vi "Configure Standard Waveform.vi"(0 "VISA resource name":refnum<visa-resource-name>, 1 "Amplitude (0.1 Vpp)":dbl=0.1, 2 "Phase Angle (0 Degree)":dbl, 5 "Channel (1: 1)":i32(ring)=1 items=["1"=1, "2"=2], 7 "Waveform Function (0: Sine)":i32(ring) items=["Sine"=0, "Square"=1, "Ramp"=2, "Noise"=3, "DC"=4, "Triangle"=5, "Pulse"=6, "Sinc"=11, "D-Lorentz"=12, "Gaussian"=13, "Expo Fall"=14, "Expo Rise"=15, "Haversine"=16], 9 "Frequency/Sample Rate/Bandwidth (1000 Hz)":dbl=1000.0 format="%#.4f", 11 "error in (no error)":errorcluster, 12 "Amplitude Unit (0: Vpp)":i32(ring) items=["Vpp", "VRMS", "DBM"], 13 "Angle Unit (0: Degree)":i32(ring) items=["Degree", "Radian", "Second"], 14 "DC Offset (0 V)":dbl) -> (4 "VISA resource name out":refnum<visa-resource-name>, 15 "error out":errorcluster)   [LabVIEW 2020, in "Agilent 3352X Series.lvlib"]
doc: "Selects a standard waveform and configure the frequency/sample rate, amplitude, offset, and phase for it.\nStandard waveform includes Sine, Square, Ramp, Noise, DC, Triangle, Sinc, D-Lorentz, Gaussian, Expo Fall, Expo Rise and Haversine\nUse Configure PRBS Waveform.vi to configure PRBS waves; use Configure Pulse Waveform.vi to configure Pulse waves.\nUse Configure Standard Waveform Advanced (Ramp) VI to set ramp symmetry for ramp wave; use Configure Standard Waveform Advanced (Suqare) VI to set duty cycle for square wave.\n<b>Note</b>:\n(1). Using this vi will automatically turn off sweep and switch to fixed frequency mode.\n(2). When select Sinc, D-Lorentz, Gaussian, Expo Fall, Expo Rise and HaverSine, a system owned Arbitrary wave is loaded and you can do arbitrary wave related settings like Filter mode and Advance mode use Configure Arbitrary Waveform (Advanced).vi"
uses:
  Agilent 3352X Series.lvlib
panel:
  # "Amplitude Settings"
  # "Phase Settings"
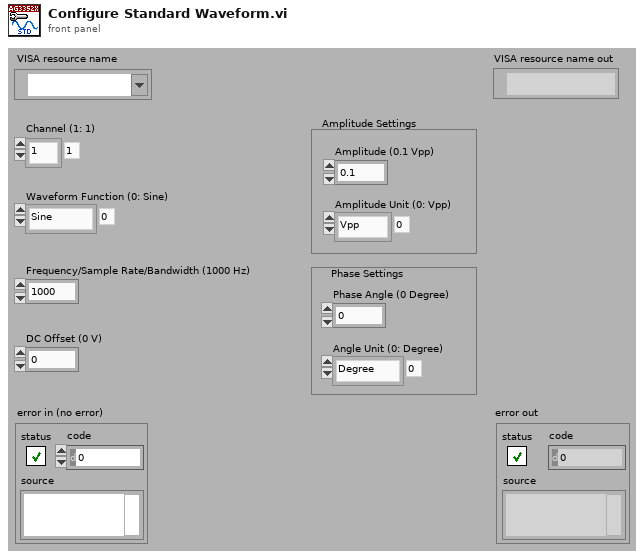
[diagram p1: front panel]
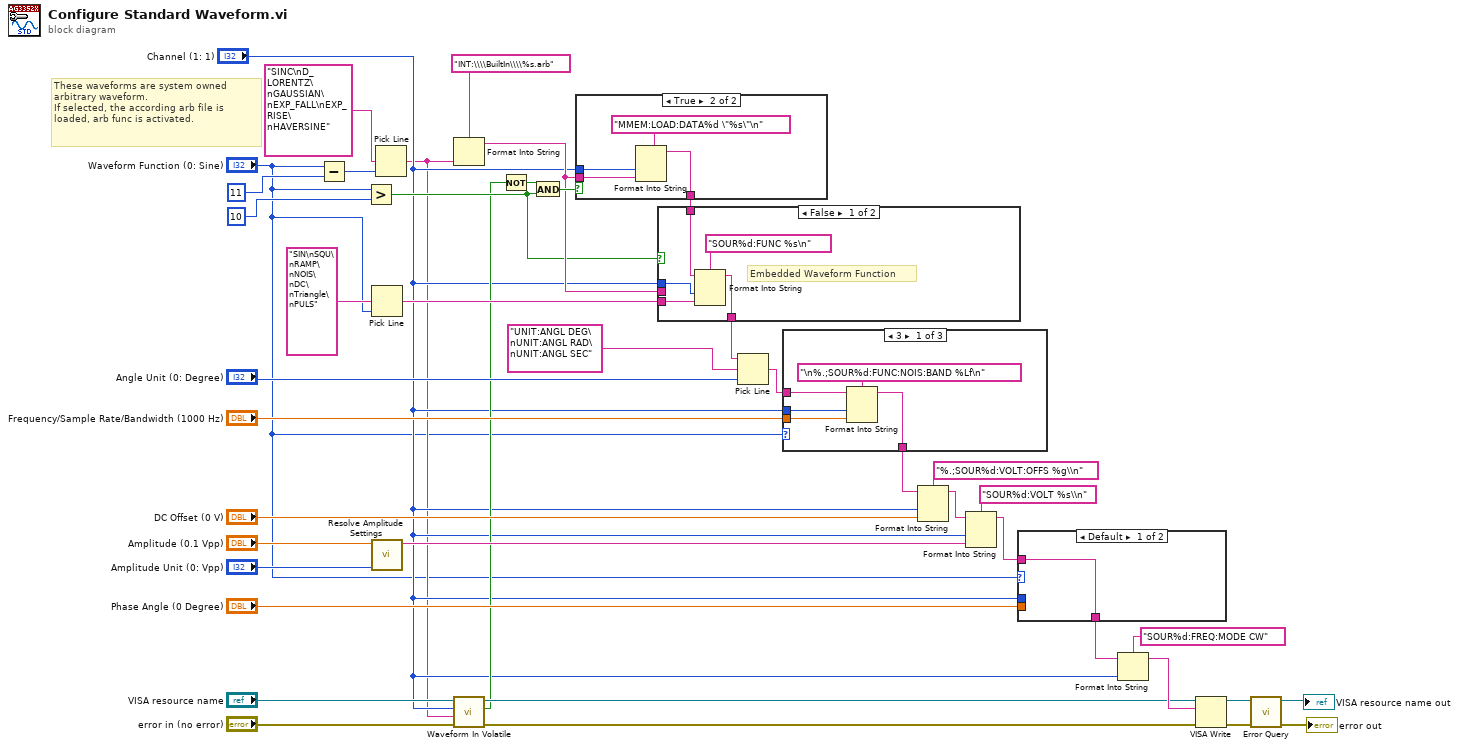
[diagram p0: block diagram]
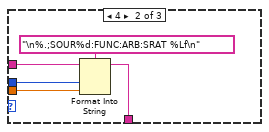
[diagram p2: hidden frame]
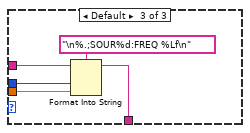
[diagram p3: hidden frame]
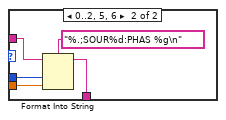
[diagram p4: hidden frame]
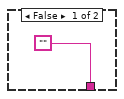
[diagram p5: hidden frame]
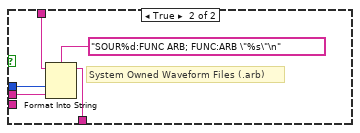
[diagram p6: hidden frame]
diagram:
  # "These waveforms are system owned arbitrary waveform.\nIf selected, the according arb file is loaded, arb func is activated."
  n1 = Subtract(x="Waveform Function (0: Sine)", y=11) -> (x-y=w27:i32)
  n2 = Greater?(x="Waveform Function (0: Sine)", y=10) -> (0:w14:bool)
  n3 = Pick Line(multi-line string="SIN\nSQU\nRAMP\nNOIS\nDC\nTriangle\nPULS", line index="Waveform Function (0: Sine)") -> (output string=w30:string)  [unwired: 1 out]
  n4 = call "Resolve Amplitude Settings.vi"("Amplitude Unit (0: VPP)"="Amplitude Unit (0: Vpp)", "Amplitude (1 Vpp)"="Amplitude (0.1 Vpp)") -> ("Resulting String"=w33:string)  [unwired: 9 out]
  n5 = Pick Line(multi-line string="SINC\nD_LORENTZ\nGAUSSIAN\nEXP_FALL\nEXP_RISE\nHAVERSINE", line index=w27) -> (output string=w4:string)  [unwired: 1 out]
  n6 = Format Into String(format string="INT:\\\\BuiltIn\\\\%s.arb", w4) -> (resulting string=w23:string)  [unwired: 2 in, 1 out]
  n7 = call "Waveform In Volatile.vi"("error in (no error)"="error in (no error)", "Arbitrary Waveform Name"=w4, "Channel (1: 1)"="Channel (1: 1)", "VISA resource name"="VISA resource name") -> ("error out"=w2:errorcluster, "Wave In Volatile?"=w6:bool, "VISA resource name out"=w7:refnum<visa-resource-name>)  [unwired: 5 out]
  n8 = Not(x=w6) -> (.not. x?=w15:bool)
  n9 = And(x=w15, y=w14) -> (x .and. y?=w26:bool)
  n10 = case shown="True" w26 {
    tunnel: "Channel (1: 1)" -> [_ w46]
    tunnel: ["" ("Empty String Constant") w45] -> w25
    tunnel: w23 -> [_ w44]
    frame False {
    }
    frame True {
      n11 = Format Into String(format string="MMEM:LOAD:DATA%d \"%s\"\n", w46, w44) -> (resulting string=w45:string)  [unwired: 2 in, 1 out]
    }
  }
  n12 = case shown="False" w14 {
    tunnel: "Channel (1: 1)" -> [w51 w56]
    tunnel: w30 -> [w50 _]
    tunnel: [w49 w54] -> w13
    tunnel: w23 -> [_ w55]
    tunnel: w25 -> [w48 w53]
    frame False {
      # "Embedded Waveform Function"
      n13 = Format Into String(format string="SOUR%d:FUNC %s\n", initial string=w48, w51, w50) -> (resulting string=w49:string)  [unwired: 1 in, 1 out]
    }
    frame True {
      # "System Owned Waveform Files (.arb)"
      n14 = Format Into String(format string="SOUR%d:FUNC ARB; FUNC:ARB \"%s\"\n", initial string=w53, w56, w55) -> (resulting string=w54:string)  [unwired: 1 in, 1 out]
    }
  }
  n15 = Pick Line(string ("")=w13, multi-line string="UNIT:ANGL DEG\nUNIT:ANGL RAD\nUNIT:ANGL SEC", line index="Angle Unit (0: Degree)") -> (output string=w17:string)
  n16 = case shown="3" "Waveform Function (0: Sine)" {
    tunnel: "Channel (1: 1)" -> [w61 w64 w71]
    tunnel: "Frequency/Sample Rate/Bandwidth (1000 Hz)" -> [w60 w63 w70]
    tunnel: [w59 w66 w69] -> w18
    tunnel: w17 -> [w58 w65 w68]
    frame 3 {
      n17 = Format Into String(format string="\n%.;SOUR%d:FUNC:NOIS:BAND %Lf\n", initial string=w58, w61, w60) -> (resulting string=w59:string)  [unwired: 1 in, 1 out]
    }
    frame 4 {
      n18 = Format Into String(format string="\n%.;SOUR%d:FUNC:ARB:SRAT %Lf\n", initial string=w65, w64, w63) -> (resulting string=w66:string)  [unwired: 1 in, 1 out]
    }
    frame Default {
      n19 = Format Into String(format string="\n%.;SOUR%d:FREQ %Lf\n", initial string=w68, w71, w70) -> (resulting string=w69:string)  [unwired: 1 in, 1 out]
    }
  }
  n20 = Format Into String(format string="%.;SOUR%d:VOLT:OFFS %g\\n", initial string=w18, "Channel (1: 1)", "DC Offset (0 V)") -> (resulting string=w39:string)  [unwired: 1 in, 1 out]
  n21 = Format Into String(format string="SOUR%d:VOLT %s\\n", initial string=w39, "Channel (1: 1)", w33) -> (resulting string=w16:string)  [unwired: 1 in, 1 out]
  n22 = case shown="Default" "Waveform Function (0: Sine)" {
    tunnel: w16 -> [w73 w77]
    tunnel: "Channel (1: 1)" -> [_ w76]
    tunnel: [w73 w75] -> w22
    tunnel: "Phase Angle (0 Degree)" -> [_ w74]
    frame Default {
    }
    frame 0..2, 5, 6 {
      n23 = Format Into String(format string="%.;SOUR%d:PHAS %g\n", initial string=w77, w76, w74) -> (resulting string=w75:string)  [unwired: 1 in, 1 out]
    }
  }
  n24 = Format Into String(format string="SOUR%d:FREQ:MODE CW", initial string=w22, "Channel (1: 1)") -> (resulting string=w21:string)  [unwired: 1 in, 1 out]
  n25 = VISA Write(VISA resource name=w7, write buffer=w21, error in (no error)=w2) -> (VISA resource name out=w37:refnum<visa-resource-name>, error out=w36:errorcluster)  [unwired: 1 out]
  n26 = call "Error Query.vi"("error in (no error)"=w36, "VISA resource name"=w37) -> ("error out"=→"error out":errorcluster, "VISA resource name out"=→"VISA resource name out":refnum<visa-resource-name>)  [unwired: 8 out]
